vi "ProdaNG.Tree.Fglb.vi"(7 "Action (add)":T3=enum."add", 8 "error in":errorcluster, 10 "entry in":T1) -> (0 "error out":errorcluster, 1 "active row":i32, 2 "found entry":T1)   [LabVIEW 2016]
uses:
  ProdaNG.Tree.Fglb.Action.ctl
  ProdaNG.Tree.Fglb.Data.ctl
  ProdaNG.Tree.Fglb.Element.ctl
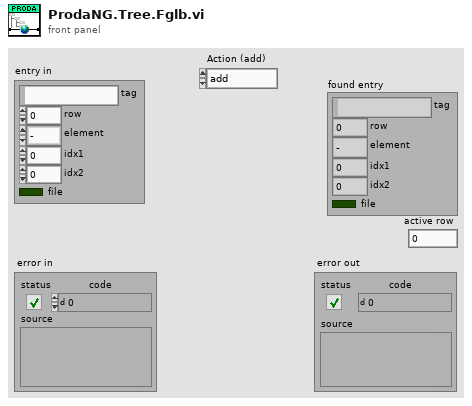
[diagram p1: front panel]
types:
  T1 = typedef "ProdaNG.Tree.Fglb.Data.ctl" = cluster{"tag":string, "row":i32, "element":T2, "idx1":i32, "idx2":i32, "file":bool}
  T2 = typedef "ProdaNG.Tree.Fglb.Element.ctl" = enum16{"-", "PP", "TS", "TP", "TV"}
  T3 = typedef "ProdaNG.Tree.Fglb.Action.ctl" = enum16{"init", "add", "get by row", "get by tag", "get by idx"}
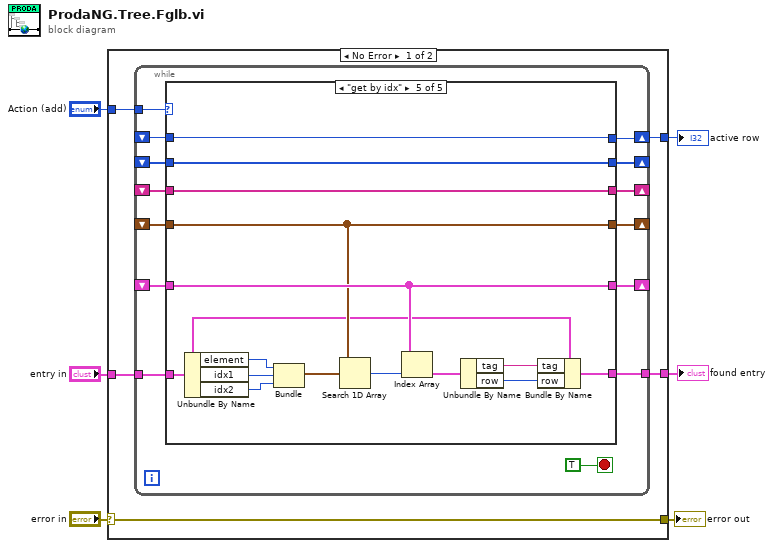
[diagram p0: block diagram]
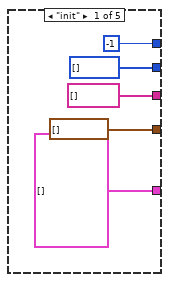
[diagram p2: hidden frame]
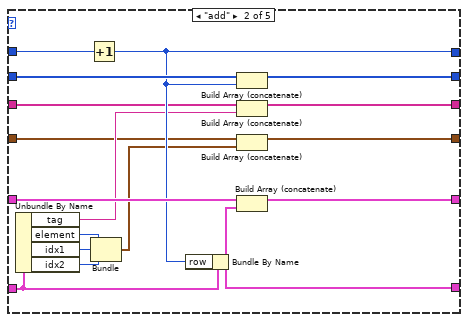
[diagram p3: hidden frame]
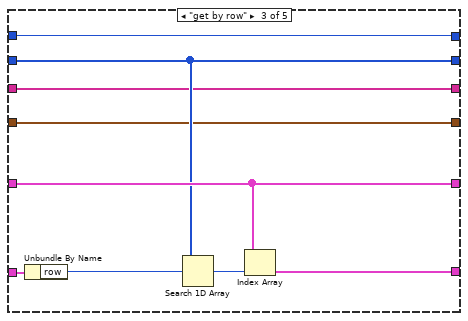
[diagram p4: hidden frame]
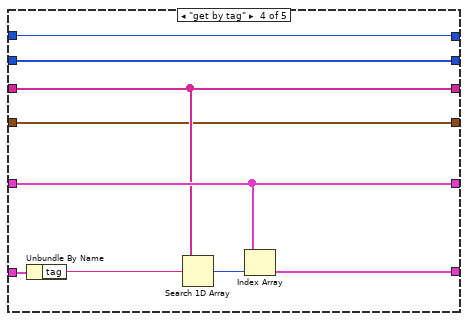
[diagram p5: hidden frame]
diagram:
  n1 = case shown="No Error" "error in" {
    selector: "error in" -> [w11 w81]
    tunnel: [w11 w81] -> w5
    tunnel: "Action (add)" -> [w10 _]
    tunnel: "entry in" -> [w9 _]
    tunnel: [w8 _] -> w3
    tunnel: [w7 _] -> w2
    frame No Error {
      n2 = while {
        tunnel: w10 -> [w25]
        tunnel: w9 -> [w24]
        shift-right: [w23] -> _
        shift-left: _ -> [w22]
        shift-right: [w21] -> _
        shift-left: _ -> [w20]
        shift-right: [w19] -> w7
        shift-left: _ -> [w18]
        tunnel: [w17] -> w8
        shift-right: [w14] -> _
        shift-left: _ -> [w15]
        shift-right: [w13] -> _
        shift-left: _ -> [w12]
        stop <- TRUE stop-if-true
        n3 = case shown="\"get by idx\"" w25 {
          tunnel: w24 -> [_ w40 w51 w60 w70]
          tunnel: [T1[] [] w44 w53 w62 w78] -> w23
          tunnel: w22 -> [_ w45 w53 w62 w78]
          tunnel: [i32[] [] w46 w52 w61 w77] -> w21
          tunnel: w20 -> [_ w47 w52 w61 w77]
          tunnel: [-1 ("row") w42 w56 w65 w80] -> w19
          tunnel: w18 -> [_ w43 w56 w65 w80]
          tunnel: [_ w41 w54 w63 w67] -> w17
          tunnel: [string[] [] w39 w49 w58 w76] -> w14
          tunnel: w15 -> [_ w38 w49 w58 w76]
          tunnel: [cluster{"element":T2, "idx1":i32, "idx2":i32}[] [] w33 w48 w57 w75] -> w13
          tunnel: w12 -> [_ w34 w48 w57 w75]
          frame "init" {
          }
          frame "add" {
            n4 = Unbundle By Name(w40) -> ("tag"=w37:string, "element"=w31:T2, "idx1"=w36:i32, "idx2"=w35:i32)
            n5 = Increment(x=w43) -> (x+1=w42:i32)
            n6 = Bundle("element"=w31, "idx1"=w36, "idx2"=w35) -> (w32:cluster{"element":T2, "idx1":i32, "idx2":i32})  [unwired: 1 in]
            n7 = Bundle By Name(cluster=w40, "row"=w42) -> (w41:T1)
            n8 = Build Array (concatenate)(w47, w42) -> (w46:i32[])
            n9 = Build Array (concatenate)(w38, w37) -> (w39:string[])
            n10 = Build Array (concatenate)(w34, w32) -> (w33:cluster{"element":T2, "idx1":i32, "idx2":i32}[])
            n11 = Build Array (concatenate)(w45, w41) -> (w44:T1[])
          }
          frame "get by row" {
            n12 = Unbundle By Name(w51) -> ("row"=w50:i32)
            n13 = Search 1D Array(1D array=w52, element=w50) -> (index of element=w55:i32)  [unwired: 1 in]
            n14 = Index Array(array=w53, index=w55) -> (element=w54:T1)
          }
          frame "get by tag" {
            n15 = Unbundle By Name(w60) -> ("tag"=w59:string)
            n16 = Search 1D Array(1D array=w58, element=w59) -> (index of element=w64:i32)  [unwired: 1 in]
            n17 = Index Array(array=w62, index=w64) -> (element=w63:T1)
          }
          frame "get by idx" {
            n18 = Unbundle By Name(w70) -> ("element"=w72:T2, "idx1"=w74:i32, "idx2"=w66:i32)
            n19 = Bundle("element"=w72, "idx1"=w74, "idx2"=w66) -> (w73:cluster{"element":T2, "idx1":i32, "idx2":i32})  [unwired: 1 in]
            n20 = Search 1D Array(1D array=w75, element=w73) -> (index of element=w79:i32)  [unwired: 1 in]
            n21 = Index Array(array=w78, index=w79) -> (element=w71:T1)
            n22 = Unbundle By Name(w71) -> ("tag"=w69:string, "row"=w68:i32)
            n23 = Bundle By Name(cluster=w70, "tag"=w69, "row"=w68) -> (w67:T1)
          }
        }
      }
    }
    frame Error {
    }
  }
  "error out" <- w5
  "active row" <- w2
  "found entry" <- w3
